vi "UI Build Tree Items.vi"(8 "error in (no error)":errorcluster, 11 "LangData in":refnum<class "Project Data.lvclass">) -> (0 "error out":errorcluster, 1 "RTM List":T2(array[cluster]), 2 "VI List":T2(array[cluster]), 3 "LangData out":refnum<class "Project Data.lvclass">, 5 "SR List":T1)   [LabVIEW 2013, in "SET Project Editor.lvlib" / "Controller.lvclass"]
uses:
  Controller.lvclass
  SET Project Data/Project Data Class/Project Data.lvclass
  SET Project Data/Project Data Class/Project Data.lvclass/Project Data.ctl
  SET Project Data/VI Class/VI Data.lvclass
  SET Project Data/Menu Class/Menu Data.lvclass/Menu Data.ctl
  SET Project Data/Menu Class/Read Menu Path (Relative).vi
  SET Project Data/Menu Class/Read Menu Item LUT.vi
  SET Project Data/Project Data Class/Read Menu Table.vi
  SET Project Data/Control Classes/GObject/Read Label.vi
  SET Project Data/Control Classes/GObject/Read ClassName.vi
  SET Project Data/Control Classes/GObject/Read UID.vi
  SET Project Data/Control Classes/GObject/Read Owning VI.vi
  SET Project Data/Control Classes/GObject/GObject.lvclass
  SET Project Data/Menu Class/Menu Data.lvclass
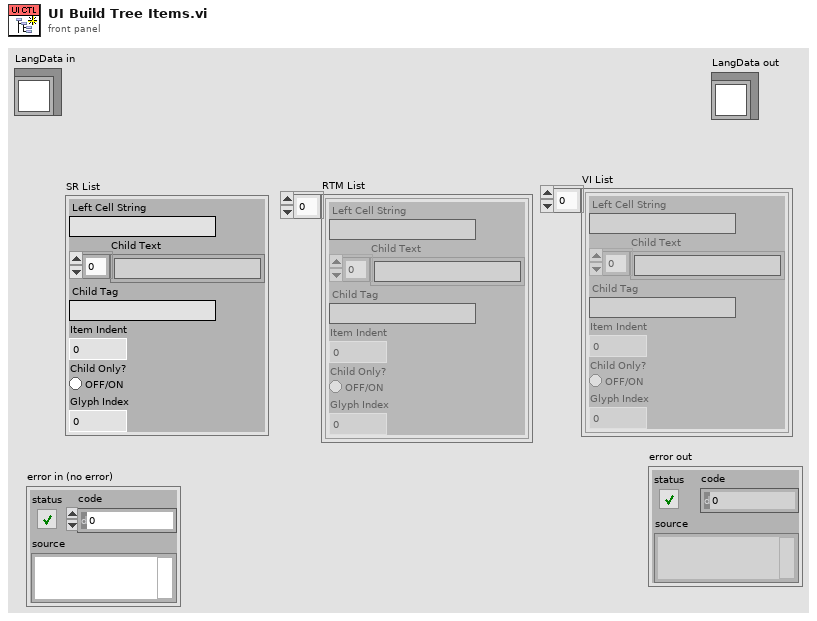
[diagram p1: front panel]
types:
  T1 = cluster{"Left Cell String":string, "Child Text":string[], "Child Tag":string, "Item Indent":i32, "Child Only?":bool, "Glyph Index":i32}
  T2 = cluster{"Left Cell String":string, "Child Text":string[], "Child Tag":string, "Item Indent":i32, "Child Only?":bool, "Glyph Index":i32}[]
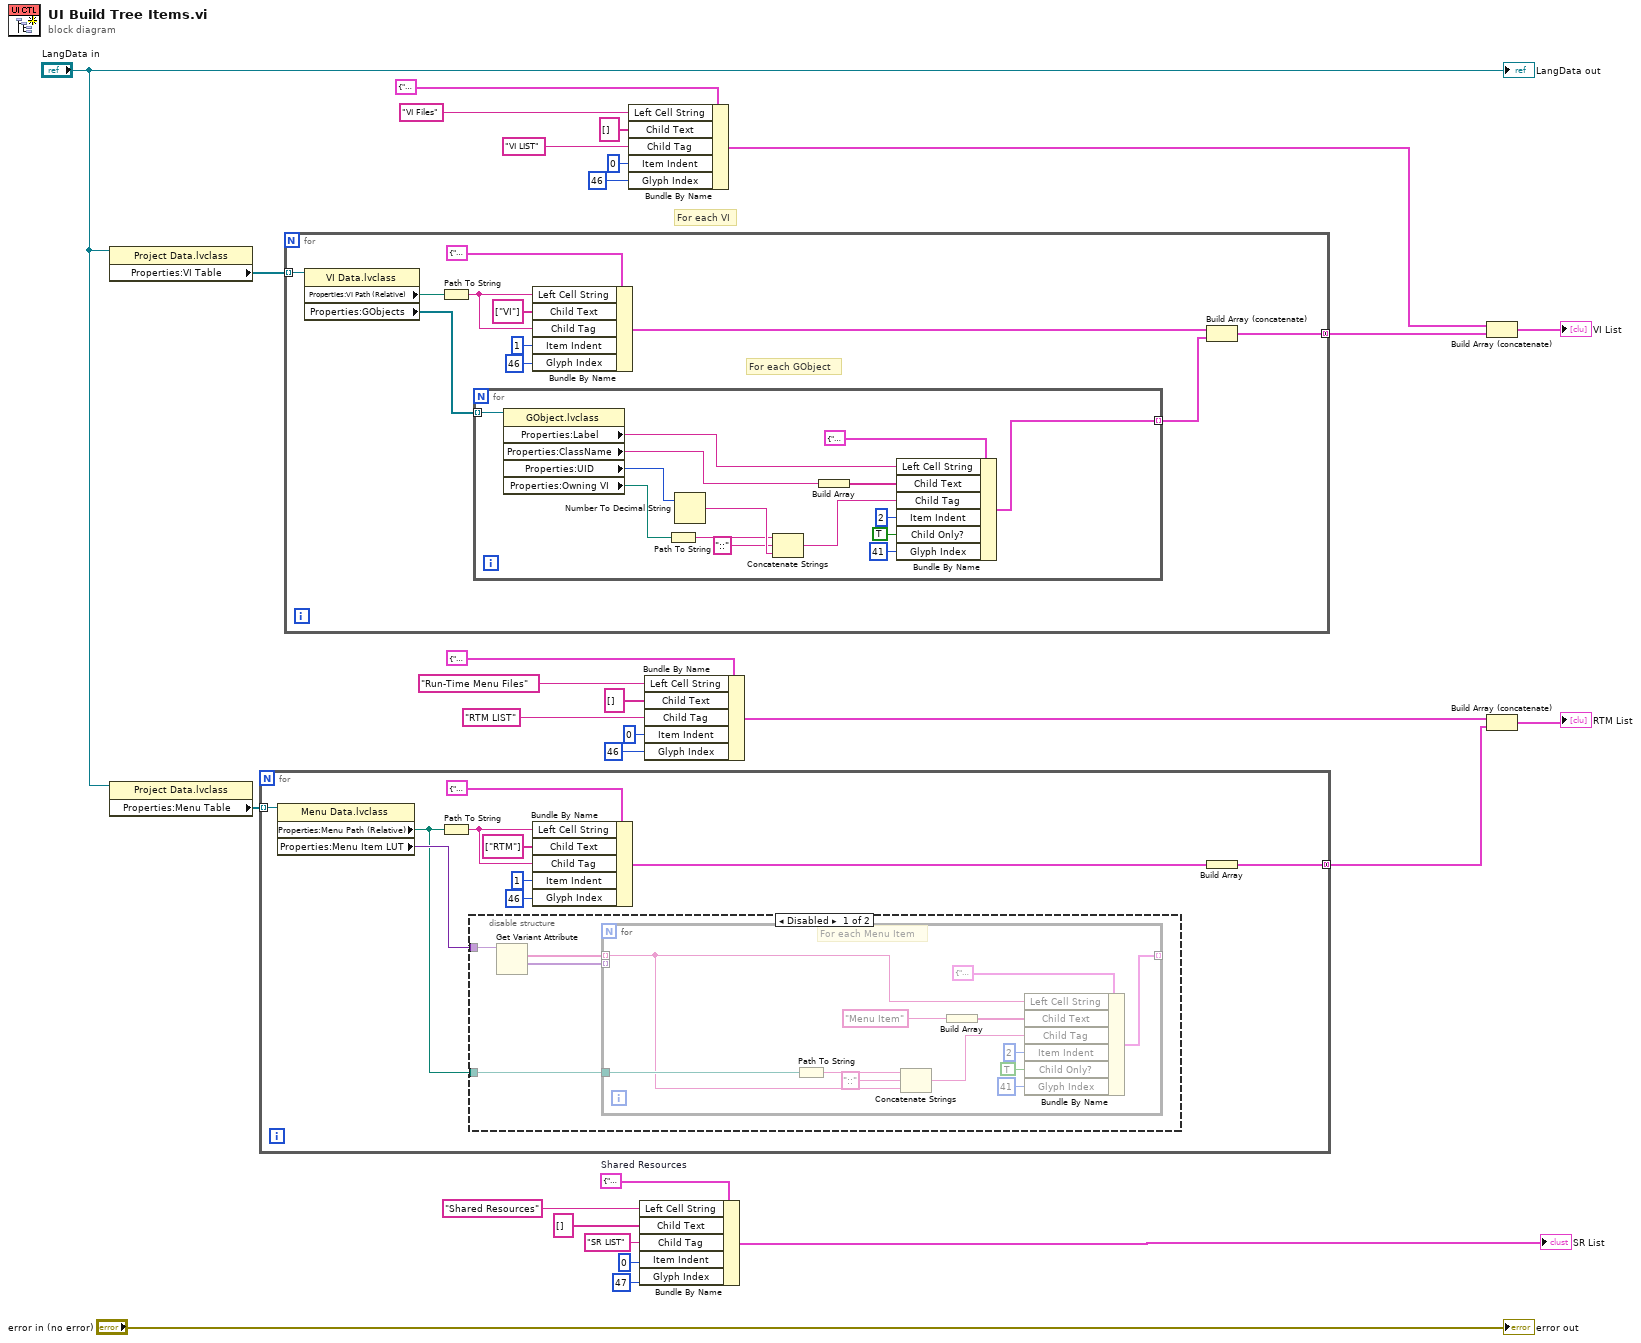
[diagram p0: block diagram]
diagram:
  w7 = T1 {"Left Cell String"="", "Child Text"=[], "Child Tag"="", "Item Indent"=0, "Child Only?"=FALSE, "Glyph Index"=0}  # Shared Resources
  # "For each VI"
  n1 = property class="Project Data.lvclass"(reference="LangData in") -> ("Properties:VI Table"=w29:refnum<class "VI Data.lvclass">[])  [unwired: 1 in, 2 out]
  n2 = property class="Project Data.lvclass"(reference="LangData in") -> ("Properties:Menu Table"=w26:refnum<class "Menu Data.lvclass">[])  [unwired: 1 in, 2 out]
  n3 = for {
    tunnel: w26 -> [w39] mode=indexing
    tunnel: [w32] -> w8 mode=concatenating
    n4 = property class="Menu Data.lvclass"(reference=w39) -> ("Properties:Menu Path (Relative)"=w30:path, "Properties:Menu Item LUT"=w31:variant)  [unwired: 1 in, 2 out]
    n5 = Path To String(path=w30) -> (string=w36:string)
    n6 = disable-structure shown="Disabled" {
      disable-tunnel: w31 -> [w43 _]
      disable-tunnel: w30 -> [w40 _]
      frame Disabled {
        n7 = Get Variant Attribute(Variant=w43) -> (names=w42:string[], values=w41:variant[])  [unwired: 3 in, 2 out]
        n8 = for {
          tunnel: [w47] -> _ mode=indexing
          tunnel: w42 -> [w44] mode=indexing
          tunnel: w41 -> [_] mode=indexing
          tunnel: w40 -> [w45]
          # "For each Menu Item"
          n9 = Path To String(path=w45) -> (string=w53:string)
          n10 = Concatenate Strings(w53, "::" ("string"), w44) -> (w55:string)
          n11 = Build Array("Menu Item") -> (w49:string[])
          n12 = Bundle By Name(cluster=T1 {"Left Cell String"="", "Child Text"=[], "Child Tag"="", "Item Indent"=0, "Child Only?"=FALSE, "Glyph Index"=0} ("Item"), "Left Cell String"=w44, "Child Text"=w49, "Child Tag"=w55, "Item Indent"=2, "Child Only?"=TRUE, "Glyph Index"=41) -> (w47:T1)
        }
      }
      frame Enabled {
      }
    }
    n13 = Bundle By Name(cluster=T1 {"Left Cell String"="", "Child Text"=[], "Child Tag"="", "Item Indent"=0, "Child Only?"=FALSE, "Glyph Index"=0} ("Item"), "Left Cell String"=w36, "Child Text"=string[] ["RTM"], "Child Tag"=w36, "Item Indent"=1, "Glyph Index"=46) -> (w33:T1)
    n14 = Build Array(w33) -> (w32:T2)
  }
  n15 = for {
    tunnel: w29 -> [w66] mode=indexing
    tunnel: [w57] -> w25 mode=concatenating
    # "For each GObject"
    n16 = property class="VI Data.lvclass"(reference=w66) -> ("Properties:VI Path (Relative)"=w65:path, "Properties:GObjects"=w59:refnum<class "GObject.lvclass">[])  [unwired: 1 in, 2 out]
    n17 = Path To String(path=w65) -> (string=w62:string)
    n18 = for {
      tunnel: w59 -> [w81] mode=indexing
      tunnel: [w67] -> w56 mode=indexing
      n19 = property class="GObject.lvclass"(reference=w81) -> ("Properties:Label"=w70:string, "Properties:ClassName"=w71:string, "Properties:UID"=w69:i32, "Properties:Owning VI"=w68:path)  [unwired: 1 in, 2 out]
      n20 = Path To String(path=w68) -> (string=w77:string)
      n21 = Number To Decimal String(number=w69) -> (decimal integer string=w79:string)  [unwired: 1 in]
      n22 = Concatenate Strings(w77, "::" ("string"), w79) -> (w80:string)
      n23 = Build Array(w71) -> (w73:string[])
      n24 = Bundle By Name(cluster=T1 {"Left Cell String"="", "Child Text"=[], "Child Tag"="", "Item Indent"=0, "Child Only?"=FALSE, "Glyph Index"=0} ("Item"), "Left Cell String"=w70, "Child Text"=w73, "Child Tag"=w80, "Item Indent"=2, "Child Only?"=TRUE, "Glyph Index"=41) -> (w67:T1)
    }
    n25 = Bundle By Name(cluster=T1 {"Left Cell String"="", "Child Text"=[], "Child Tag"="", "Item Indent"=0, "Child Only?"=FALSE, "Glyph Index"=0} ("Item"), "Left Cell String"=w62, "Child Text"=string[] ["VI"], "Child Tag"=w62, "Item Indent"=1, "Glyph Index"=46) -> (w58:T1)
    n26 = Build Array (concatenate)(w58, w56) -> (w57:T2)
  }
  n27 = Bundle By Name(cluster=T1 {"Left Cell String"="", "Child Text"=[], "Child Tag"="", "Item Indent"=0, "Child Only?"=FALSE, "Glyph Index"=0} ("Item"), "Left Cell String"="VI Files", "Child Text"=string[] [], "Child Tag"="VI LIST", "Item Indent"=0, "Glyph Index"=46) -> (w18:T1)
  n28 = Bundle By Name(cluster=w7, "Left Cell String"="Shared Resources", "Child Text"=string[] [], "Child Tag"="SR LIST", "Item Indent"=0, "Glyph Index"=47) -> (→"SR List":T1)
  n29 = Bundle By Name(cluster=T1 {"Left Cell String"="", "Child Text"=[], "Child Tag"="", "Item Indent"=0, "Child Only?"=FALSE, "Glyph Index"=0} ("Item"), "Left Cell String"="Run-Time Menu Files", "Child Text"=string[] [], "Child Tag"="RTM LIST", "Item Indent"=0, "Glyph Index"=46) -> (w10:T1)
  n30 = Build Array (concatenate)(w18, w25) -> (→"VI List":T2)
  n31 = Build Array (concatenate)(w10, w8) -> (→"RTM List":T2)
  "error out" <- "error in (no error)"
  "LangData out" <- "LangData in"
